vi "ConditioningState.vi"() -> ()   [LabVIEW 2014]
uses:
  ParamsArray.ctl
  state.lvsc/State.ctl
  Licker.lvclass
  Juicer.lvclass
  Acquisition.lvclass
  <vilib>/Utility/error.llb/DialogType.ctl
  Stimulus.lvclass
  state.lvsc/Inputs.ctl
  state.lvsc/Trigger.ctl
  <vilib>/Statechart/Common/IntGuid.ctl
  <vilib>/Statechart/Common/DbgID.ctl
  state.lvsc/StatechartState.ctl
  <vilib>/Utility/file.llb/Read From Spreadsheet File (DBL).vi
  state.lvsc/CompanionDiagram.vi/43/SC Main.vi
  <vilib>/Statechart/Nodes/EventFiring/NI_SC_EventFiringNode.xnode
  state.lvsc
  <vilib>/Statechart/Infrastructure/RTStatechart/RunTime SCN.xnode
  state.lvsc/Outputs.ctl
  <vilib>/Statechart/Common/NI_SC_LVSCCommonFiles.lvlib
panel:
  in  "default pulse duration":dbl
  in  "Local\nDatabase":bool
  in  "Que mail":dbl=500.0
  in  "mail":bool=TRUE
  in  "Reset":bool
  out "error out":errorcluster
  in  "liquid":string(combo)="water"
  in  "Thr":dbl[](array[numeric])=[10.0, 10.0, 10.0, 10.0, 10.0]
  out "Optical traces":waveform(dbl)[](graph)
  in  "Task":dbl[](array[numeric])=[0.0, 0.0, 0.0, 0.0, 0.0]
  out "Licks 2":bool[](array[boolean])
  in  "screen_setup":u16(ring) items=["Default", "1"]
  out "queue#":i32
  in  "Probes":enum16{"Testing", "1-5", "6-10"}(ring)
  in  "Display":bool
  out "Mon params":dbl[][](array[numeric])=[[100.0, 100.0, 0.0, 0.0], [100.0, 100.0, 100.0, 0.0], [100.0, 100.0, 200.0, 0.0], [100.0, 100.0, 300.0, 0.0], [100.0, 100.0, 400.0, 0.0]]
  out "Air":bool[](array[boolean])
  out "CS":bool[](array[boolean])
  out "Active States":T1[][](array[typedef])
  out "Number of Licks":dbl[](array[numeric]) caption="#Licks"
  in  "LICK":bool[](array[boolean])=[FALSE, FALSE, FALSE, FALSE, FALSE]
  out "Elapsed Time":dbl[](array[numeric]) caption="Time"
  out "Rewards Given":dbl[](array[numeric]) caption="#Rew"
  out "Water":bool[](array[boolean])
  out "Licks":bool[](array[boolean])
  out "Sti":i32
  in  "RUN":bool[](array[boolean])=[FALSE, FALSE, FALSE, FALSE, FALSE]
  out "Lick":i32
  out "Acq":i32
  out "Jui":i32
  in  "REC":bool[](array[boolean])=[FALSE, FALSE, FALSE, FALSE, FALSE]
  in  "Stop":bool
  in  "Params":T2={"Mice ID"=[1.0, 1.0, 1.0, 1.0, 1.0], "ExpType"=["Orientation", "Orientation", "Orientation", "Orientation", "Orientation"], "Trial Interval"=[30.0, 30.0, 30.0, 30.0, 30.0], "Pulse Duration"=[158.0, 152.0, 156.0, 167.0, 172.0], "microL_per_pulse"=[6.0, 6.0, 6.0, 6.0, 6.0], "Response Interval"=[1000.0, 1000.0, 1000.0, 1000.0, 1000.0], "Bad Delay"=[180.0, 180.0, 180.0, 180.0, 180.0], "Response Period"=[30.0, 30.0, 30.0, 30.0, 30.0], "liquid_type"="water", "Stimuli"=["", "", "", "", ""], "Rewarded Stimuli"=["", "", "", "", ""], "AirDur"=[400.0, 400.0, 400.0, 400.0, 400.0]} {"AirDur" format="%#_13g"}
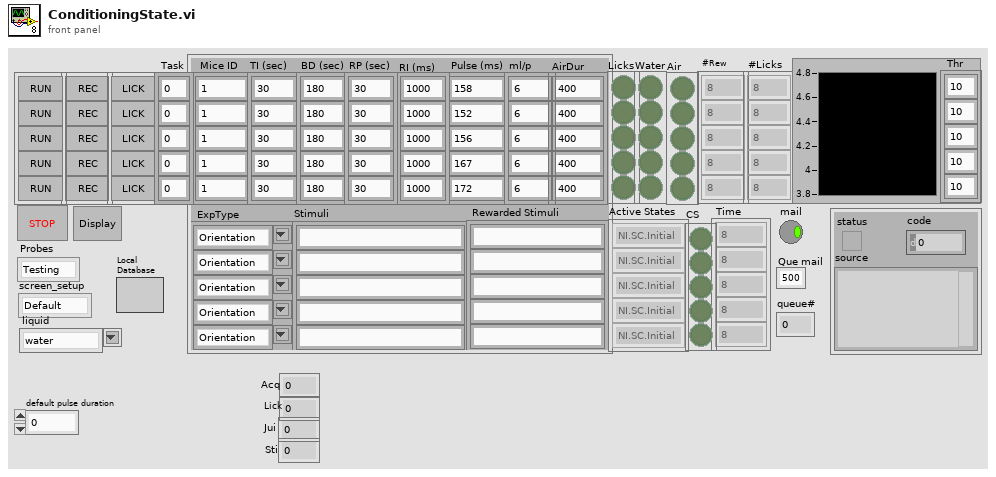
[diagram p1: front panel]
types:
  T1 = typedef "state.lvsc/State.ctl" = enum16{"NI.SC.Initial", "NI.SC.History", "NI.SC.ShallowHistory", "NI.SC.Terminal", "Reward", "Punishment", "Response \nPeriod", "EndTrial", "Start trial"}
  T2 = typedef "ParamsArray.ctl" = cluster{"Mice ID":dbl[], "ExpType":string[], "Trial Interval":dbl[], "Pulse Duration":dbl[], "microL_per_pulse":dbl[], "Response Interval":dbl[], "Bad Delay":dbl[], "Response Period":dbl[], "liquid_type":string, "Stimuli":string[], "Rewarded Stimuli":string[], "AirDur":dbl[]}
  T3 = typedef "DialogType.ctl" = u16
  T4 = typedef "Semaphore RefNum" = refnum<k1>
  T5 = enum16{"air_delivery", "beh_session", "stim_periods", "licks", "liquid_delivery", ""}
  T6 = enum16{"Get Time", "Get Elapsed Time", "Reset Elapsed Time"}
  T7 = typedef "state.lvsc/Inputs.ctl" = cluster{"Acquisition.lvclass":refnum<class "Acquisition.lvclass">, "Stimulus.lvclass":refnum<class "Stimulus.lvclass">, "Juicer.lvclass":refnum<class "Juicer.lvclass">, "Index":dbl, "error in (no error)":errorcluster, "Lick":bool, "State":string}
  T8 = typedef "state.lvsc/Trigger.ctl" = enum16{"NULL", "Lick", "Exit"}
  T9 = typedef "state.lvsc/StatechartState.ctl" = T1[]
  T10 = typedef "NI_SC_LVSCCommonFiles.lvlib/IntGuid.ctl" = cluster{"Data1":u32, "Data2":u16, "Data3":u16, "Data4":u8, "Data5":u8, "Data6":u8, "Data11":u8, "Data9":u8, "Data10":u8, "Data8":u8, "Data7":u8}
  T11 = typedef "NI_SC_LVSCCommonFiles.lvlib/DbgID.ctl" = cluster{"VIRef":u32, "IntGUID":T10}
  T12 = typedef "state.lvsc/Outputs.ctl" = cluster{"Stimulus.lvclass":refnum<class "Stimulus.lvclass">, "error out":errorcluster, "State":string, "Index":dbl, "Correct Response":bool}
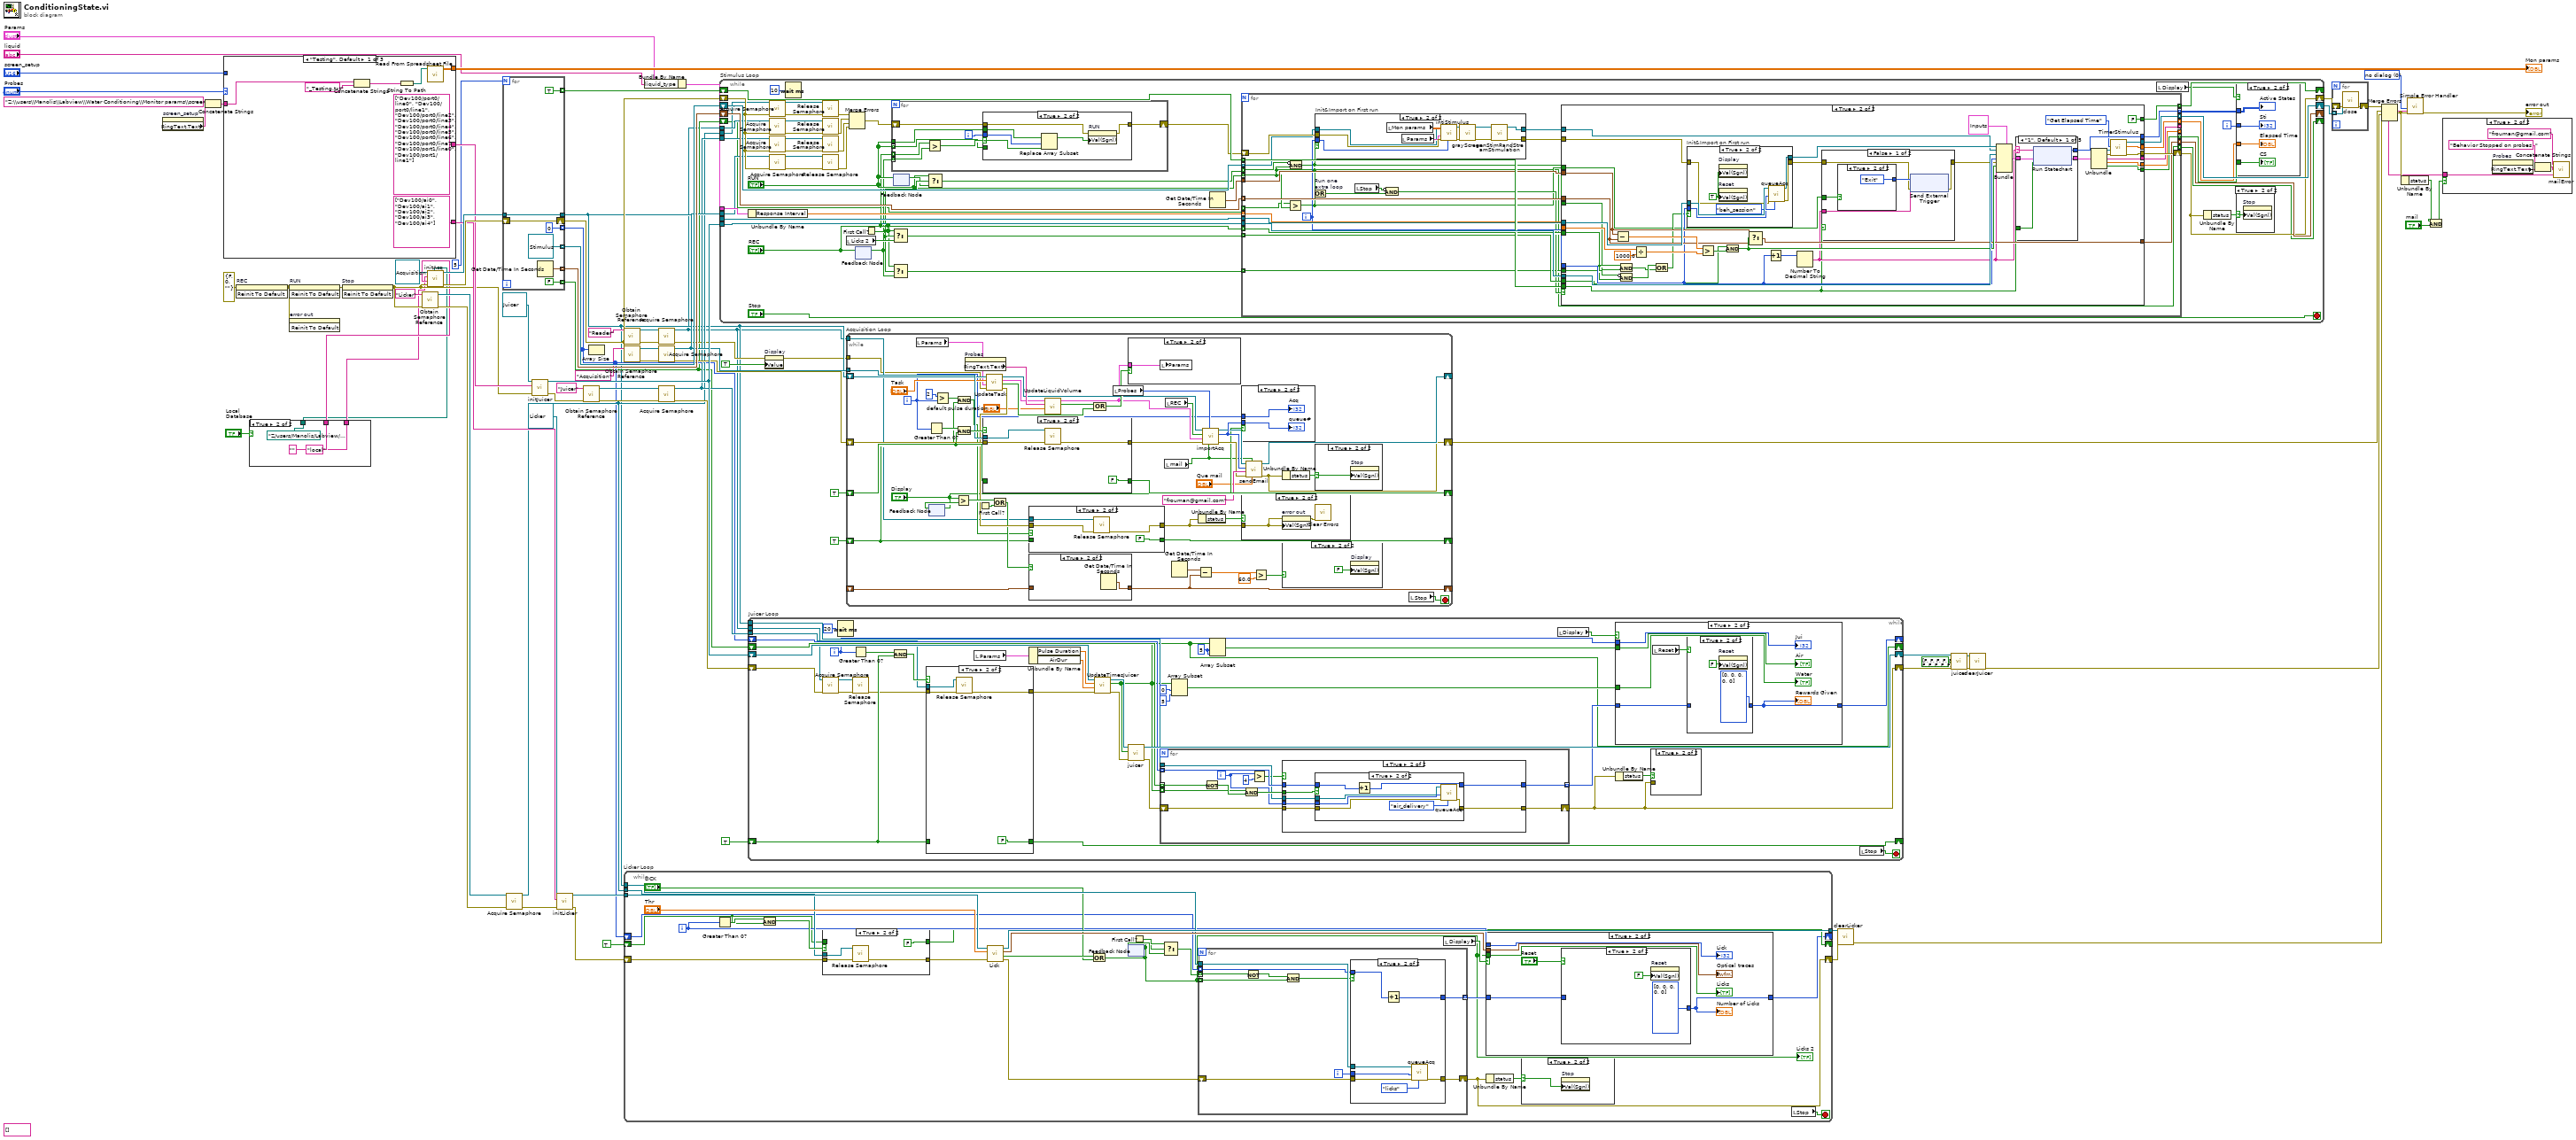
[diagram p0: block diagram]
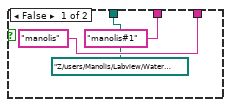
[diagram p2: hidden frame]
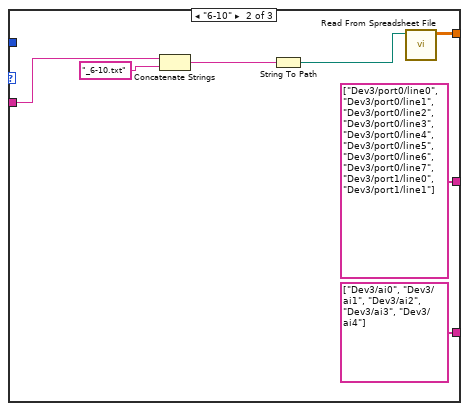
[diagram p4: hidden frame]
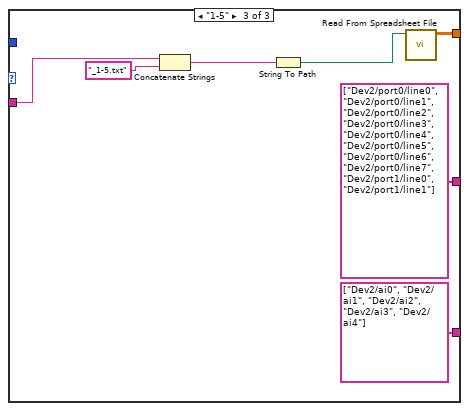
[diagram p5: hidden frame]
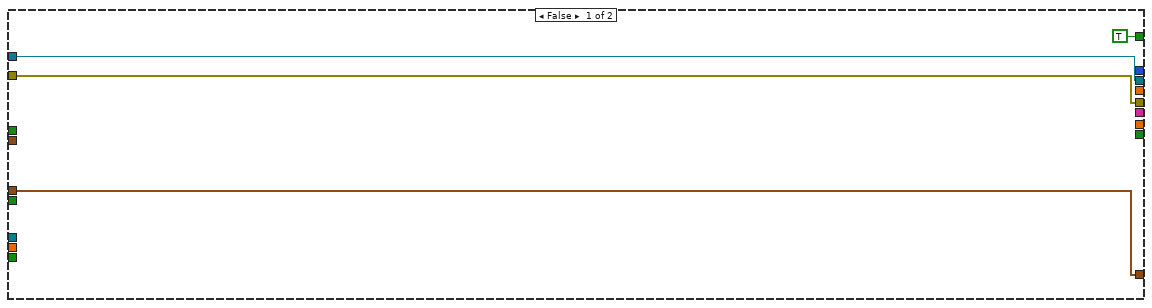
[diagram p10: hidden frame]
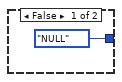
[diagram p11: hidden frame]
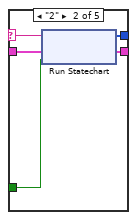
[diagram p14: hidden frame]
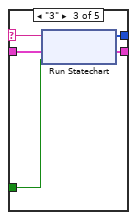
[diagram p15: hidden frame]
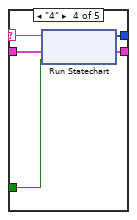
[diagram p16: hidden frame]
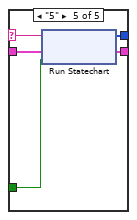
[diagram p17: hidden frame]
diagram:
  (unwired) string[] [] ("Mail addresses")
  w19 = T3 0 items=["no dialog", "OK message", "continue or stop message", "OK message + warnings", "continue/stop + warnings"] ("type of dialog (OK msg:1)")
  n1 = property on="screen_setup" class="Ring (strict)"() -> ("RingText.Text"=w49:string)  [unwired: 2 in, 2 out]
  n2 = Concatenate Strings("Z:\\users\\Manolis\\Labview\\Water Conditioning\\Monitor params\\screen_" ("file path (dialog if empty)"), w49) -> (w48:string)
  n3 = case shown="\"Testing\", Default" "Probes" {
    tunnel: [w83 w90 w97] -> w61
    tunnel: [string[] ["Dev100/port0/line0", "Dev100/port0/line1", "Dev100/port0/line2", "Dev100/port0/line3", "Dev100/port0/line4", "Dev100/port0/line5", "Dev100/port0/line6", "Dev100/port0/line7", "Dev100/port1/line0", "Dev100/port1/line1"] ("Lines") string[] ["Dev3/port0/line0", "Dev3/port0/line1", "Dev3/port0/line2", "Dev3/port0/line3", "Dev3/port0/line4", "Dev3/port0/line5", "Dev3/port0/line6", "Dev3/port0/line7", "Dev3/port1/line0", "Dev3/port1/line1"] ("Lines") string[] ["Dev2/port0/line0", "Dev2/port0/line1", "Dev2/port0/line2", "Dev2/port0/line3", "Dev2/port0/line4", "Dev2/port0/line5", "Dev2/port0/line6", "Dev2/port0/line7", "Dev2/port1/line0", "Dev2/port1/line1"] ("Lines")] -> w60
    tunnel: [string[] ["Dev100/ai0", "Dev100/ai1", "Dev100/ai2", "Dev100/ai3", "Dev100/ai4"] ("Lines") string[] ["Dev3/ai0", "Dev3/ai1", "Dev3/ai2", "Dev3/ai3", "Dev3/ai4"] ("Lines") string[] ["Dev2/ai0", "Dev2/ai1", "Dev2/ai2", "Dev2/ai3", "Dev2/ai4"] ("Lines")] -> w59
    tunnel: "screen_setup" -> [_ _ _]
    tunnel: w48 -> [w85 w91 w98]
    frame "Testing", Default {
      n4 = Concatenate Strings(w85, "_Testing.txt" ("string")) -> (w86:string)
      n5 = String To Path(string=w86) -> (path=w87:path)
      n6 = call-poly <vilib>:"Read From Spreadsheet File.vi"("file path (dialog if empty)"=w87) -> ("all rows"=w83:dbl[][])  [unwired: 6 in, 4 out]
    }
    frame "6-10" {
      n7 = Concatenate Strings(w91, "_6-10.txt" ("string")) -> (w93:string)
      n8 = String To Path(string=w93) -> (path=w94:path)
      n9 = call-poly <vilib>:"Read From Spreadsheet File.vi"("file path (dialog if empty)"=w94) -> ("all rows"=w90:dbl[][])  [unwired: 6 in, 4 out]
    }
    frame "1-5" {
      n10 = Concatenate Strings(w98, "_1-5.txt" ("string")) -> (w100:string)
      n11 = String To Path(string=w100) -> (path=w101:path)
      n12 = call-poly <vilib>:"Read From Spreadsheet File.vi"("file path (dialog if empty)"=w101) -> ("all rows"=w97:dbl[][])  [unwired: 6 in, 4 out]
    }
  }
  "Mon params" <- w61
  n13 = invoke on="REC" class="Arr (strict)" method="Reinit To Default"(error in=errorcluster {"status"=FALSE, "code"=0, "source"=""} ("error in (no error)")) -> (error out=w12:errorcluster)  [unwired: 2 in, 2 out]
  n14 = case shown="True" "Local\nDatabase" {
    tunnel: ["manolis#1" ("password") "" ("password")] -> w4
    tunnel: ["manolis" ("userID") "local" ("userID")] -> w3
    tunnel: [path "Z:/users/Manolis/Labview/Water Conditioning/sessions_remote.dsn" ("Session") path "Z:/users/Manolis/Labview/Water Conditioning/sessions_loca.dsn" ("Session")] -> w2
    frame False {
    }
    frame True {
    }
  }
  n15 = invoke on="RUN" class="Arr (strict)" method="Reinit To Default"(error in=w12) -> (error out=w71:errorcluster)  [unwired: 2 in, 2 out]
  n16 = invoke on="error out" class="Clust (strict)" method="Reinit To Default"(error in=w12) -> ()  [unwired: 2 in, 3 out]
  n17 = invoke on="Stop" class="Bool (strict)" method="Reinit To Default"(error in=w71) -> (error out=w29:errorcluster)  [unwired: 2 in, 2 out]
  n18 = call <vilib>:"Obtain Semaphore Reference.vi"("error in (no error)"=w29, "name (unnamed)"="Licker") -> ("error out"=w32:errorcluster, "semaphore"=w30:T4)  [unwired: 3 in, 1 out]
  n19 = call-dynamic "initAcq.vi"("Session"=w2, "error in (no error)"=w29, "password"=w4, "userID"=w3, "Acquisition in"=refnum<class "Acquisition.lvclass"> refnum ("Acquisition.lvclass")) -> ("error out"=w63:errorcluster, "Acquisition out"=w64:refnum<class "Acquisition.lvclass">)  [unwired: 5 in]
  n20 = for {
    N: 5 -> [_]
    tunnel: [refnum<class "Stimulus.lvclass"> refnum ("Stimulus.lvclass")] -> w69 mode=indexing
    shift-right: [w110] -> w34
    shift-left: w63 -> [w110]
    tunnel: [TRUE] -> w65 mode=indexing
    tunnel: [FALSE] -> w17 mode=indexing
    tunnel: [0] -> w22 mode=indexing
    tunnel: [w113] -> w57 mode=indexing
    tunnel: w64 -> [w112]
    tunnel: [w112] -> w16
    n21 = Get Date/Time In Seconds() -> (seconds since 1Jan1904=w113:timestamp)
  }
  n22 = call <vilib>:"Acquire Semaphore.vi"("error in (no error)"=w32, "semaphore"=w30) -> ("error out"=w28:errorcluster, "semaphore out"=w25:T4)  [unwired: 3 in, 1 out]
  n23 = call-dynamic "initJuicer.vi"("error in (no error)"=w29, "Lines"=w60, "Juicer in"=refnum<class "Juicer.lvclass"> refnum ("Juicer.lvclass")) -> ("error out"=w41:errorcluster, "Juicer out"=w72:refnum<class "Juicer.lvclass">)  [unwired: 7 in]
  n24 = call-dynamic "initLicker.vi"("error in (no error)"=w28, "Lines"=w59, "Licker in"=refnum<class "Licker.lvclass"> refnum ("Licker.lvclass")) -> ("error out"=w78:errorcluster, "Licker out"=w80:refnum<class "Licker.lvclass">)  [unwired: 7 in]
  n25 = call <vilib>:"Obtain Semaphore Reference.vi"("error in (no error)"=w41, "name (unnamed)"="Juicer") -> ("error out"=w44:errorcluster, "semaphore"=w42:T4)  [unwired: 3 in, 1 out]
  n26 = Array Size(array=w22) -> ()  [unwired: 1 out]
  n27 = call <vilib>:"Obtain Semaphore Reference.vi"("error in (no error)"=w34, "name (unnamed)"="Reader") -> ("error out"=w45:errorcluster, "semaphore"=w47:T4)  [unwired: 3 in, 1 out]
  n28 = call <vilib>:"Obtain Semaphore Reference.vi"("error in (no error)"=w34, "name (unnamed)"="Acquisition") -> ("error out"=w37:errorcluster, "semaphore"=w35:T4)  [unwired: 3 in, 1 out]
  n29 = while "Licker Loop" {
    tunnel: w80 -> [w142]
    tunnel: [w141] -> w79
    shift-right: [w117] -> _
    shift-left: w22 -> [w123]
    tunnel: w16 -> [w135]
    tunnel: w25 -> [w129]
    shift-right: [w125] -> _
    shift-left: TRUE -> [w124]
    shift-right: [w118] -> w76
    shift-left: w78 -> [w127]
    i -> [w128]
    stop <- w143 stop-if-true
    n30 = Greater Than 0?(x=w128) -> (x > 0?=w130:bool)
    n31 = And(x=w130, y=w124) -> (x .and. y?=w131:bool)
    n32 = case shown="True" w131 {
      tunnel: [w145 FALSE] -> w125
      tunnel: w127 -> [w144 w148]
      tunnel: w124 -> [w145 _]
      tunnel: w129 -> [_ w147]
      tunnel: [w144 w146] -> w126
      frame False {
      }
      frame True {
        n33 = call <vilib>:"Release Semaphore.vi"("error in (no error)"=w148, "semaphore"=w147) -> ("error out"=w146:errorcluster)  [unwired: 4 in, 1 out]
      }
    }
    n34 = call-dynamic "Lick.vi"("error in (no error)"=w126, "% decrease Thr"="Thr", "Licker in"=w142) -> ("error out"=w138:errorcluster, "Lick?"=w136:bool[], "data"=w140:waveform(dbl)[], "Licker out"=w141:refnum<class "Licker.lvclass">)  [unwired: 5 in]
    n35 = Or(x=w136, y="LICK") -> (x .or. y?=w121:bool[])
    "Licks 2" <- w121
    n36 = feedback-in #1(w121) -> ()
    n37 = feedback #1() -> (w122:bool[])  [unwired: 1 in]
    n38 = First Call?() -> (First Call?: T/F=w120:bool)
    n39 = Select(t=w121, s=w120, f=w122) -> (s? t:f=w119:bool[])
    n40 = for {
      tunnel: w121 -> [w166] mode=indexing
      shift-right: [w169] -> w118
      shift-left: w138 -> [w170]
      tunnel: w119 -> [w165] mode=indexing
      tunnel: w123 -> [w162] mode=indexing
      tunnel: [w161] -> w132 mode=indexing
      tunnel: w135 -> [w168]
      i -> [w167]
      n41 = Not(x=w165) -> (.not. x?=w164:bool)
      n42 = And(x=w164, y=w166) -> (x .and. y?=w163:bool)
      n43 = case shown="True" w163 {
        tunnel: w167 -> [_ w176]
        tunnel: w170 -> [w172 w179]
        tunnel: [w172 w178] -> w169
        tunnel: w168 -> [_ w177]
        tunnel: w162 -> [w171 w175]
        tunnel: [w171 w174] -> w161
        frame False {
        }
        frame True {
          n44 = Increment(x=w175) -> (x+1=w174:i32)
          n45 = call-dynamic "queueAcq.vi"("table"=T5."licks", "error in (no error)"=w179, "Window Number (0...15)"=w176, "Acquisition in"=w177) -> ("error out"=w178:errorcluster)  [unwired: 5 in, 2 out]
        }
      }
    }
    n46 = local read "Display"() -> (w133:bool)
    n47 = case shown="True" w133 {
      tunnel: w140 -> [_ w156]
      tunnel: w128 -> [_ w155]
      tunnel: w132 -> [w150 w153]
      tunnel: w121 -> [_ w154]
      tunnel: [w150 w152] -> w117
      frame False {
      }
      frame True {
        n48 = case shown="True" "Reset" {
          tunnel: w153 -> [w157 _]
          tunnel: [w157 i32[] [0, 0, 0, 0, 0]] -> w152
          frame False {
          }
          frame True {
            n49 = property on="Reset" class="Bool (strict)"("Val(Sgnl)"=FALSE ("Value (Signaling)")) -> ()  [unwired: 2 in, 2 out]
          }
        }
        "Number of Licks" <- w152
        "Optical traces" <- w156
        "Lick" <- w155
        "Licks" <- w154
      }
    }
    n50 = Unbundle By Name(w118) -> ("status"=w137:bool)
    n51 = case shown="True" w137 {
      selector: w137 -> [_ w160]
      frame False {
      }
      frame True {
        n52 = property on="Stop" class="Bool (strict)"("Val(Sgnl)"=w160) -> ()  [unwired: 2 in, 2 out]
      }
    }
    n53 = local read "Stop"() -> (w143:bool)
  }
  n54 = Bundle By Name(cluster="Params", "liquid_type"="liquid") -> (w14:T2)
  n55 = call <vilib>:"Acquire Semaphore.vi"("error in (no error)"=w45, "semaphore"=w47) -> ("error out"=w23:errorcluster, "semaphore out"=w11:T4)  [unwired: 3 in, 1 out]
  n56 = call <vilib>:"Acquire Semaphore.vi"("error in (no error)"=w37, "semaphore"=w35) -> ("error out"=w33:errorcluster, "semaphore out"=w27:T4)  [unwired: 3 in, 1 out]
  n57 = call <vilib>:"Acquire Semaphore.vi"("error in (no error)"=w44, "semaphore"=w42) -> ("error out"=w40:errorcluster, "semaphore out"=w26:T4)  [unwired: 3 in, 1 out]
  n58 = while "Stimulus Loop" {
    tunnel: w72 -> [w229]
    shift-right: [w224] -> w68
    shift-left: w69 -> [w218]
    tunnel: w16 -> [w226]
    shift-right: [w225] -> _
    shift-left: w65 -> [w192]
    shift-right: [w222] -> _
    shift-left: w57 -> [w217]
    tunnel: w14 -> [w221]
    tunnel: w27 -> [w198]
    tunnel: w26 -> [w197]
    tunnel: w11 -> [w196]
    tunnel: w25 -> [w195]
    shift-right: [w182] -> w67
    shift-left: w34 -> [w203]
    shift-right: [w181] -> _
    shift-left: w17 -> [w180]
    i -> [w213]
    stop <- "Stop" stop-if-true
    n59 = Unbundle By Name(w221) -> ("Response Interval"=w219:dbl[])
    n60 = call <vilib>:"Acquire Semaphore.vi"("error in (no error)"=w203, "semaphore"=w195) -> ("error out"=w210:errorcluster, "semaphore out"=w211:T4)  [unwired: 3 in, 1 out]
    n61 = call <vilib>:"Acquire Semaphore.vi"("error in (no error)"=w203, "semaphore"=w196) -> ("error out"=w209:errorcluster, "semaphore out"=w208:T4)  [unwired: 3 in, 1 out]
    n62 = call <vilib>:"Acquire Semaphore.vi"("error in (no error)"=w203, "semaphore"=w197) -> ("error out"=w206:errorcluster, "semaphore out"=w207:T4)  [unwired: 3 in, 1 out]
    n63 = call <vilib>:"Acquire Semaphore.vi"("error in (no error)"=w203, "semaphore"=w198) -> ("error out"=w205:errorcluster, "semaphore out"=w204:T4)  [unwired: 3 in, 1 out]
    n64 = Wait (ms)(milliseconds to wait=u32 10) -> ()  [unwired: 1 out]
    n65 = call <vilib>:"Release Semaphore.vi"("error in (no error)"=w210, "semaphore"=w211) -> ("error out"=w202:errorcluster)  [unwired: 4 in, 1 out]
    n66 = call <vilib>:"Release Semaphore.vi"("error in (no error)"=w209, "semaphore"=w208) -> ("error out"=w201:errorcluster)  [unwired: 4 in, 1 out]
    n67 = call <vilib>:"Release Semaphore.vi"("error in (no error)"=w206, "semaphore"=w207) -> ("error out"=w200:errorcluster)  [unwired: 4 in, 1 out]
    n68 = call <vilib>:"Release Semaphore.vi"("error in (no error)"=w205, "semaphore"=w204) -> ("error out"=w199:errorcluster)  [unwired: 4 in, 1 out]
    n69 = local read "Licks 2"() -> (w191:bool[])
    n70 = Merge Errors(w202, w201, w200, w199) -> (w184:errorcluster)
    n71 = feedback #2() -> (w185:bool[])  [unwired: 1 in]
    n72 = feedback-in #2("REC") -> ()
    n73 = First Call?() -> (First Call?: T/F=w190:bool)
    n74 = for {
      tunnel: "RUN" -> [w236] mode=indexing
      tunnel: "RUN" -> [w235]
      tunnel: "REC" -> [w233] mode=indexing
      tunnel: w185 -> [w232] mode=indexing
      shift-right: [w230] -> w183
      shift-left: w184 -> [w231]
      i -> [w234]
      n75 = Greater?(x=w233, y=w232) -> (0:w237:bool)
      n76 = case shown="True" w237 {
        selector: w237 -> [_ w242]
        tunnel: w236 -> [_ _]
        tunnel: w235 -> [_ w244]
        tunnel: w234 -> [_ w243]
        tunnel: w231 -> [w238 w240]
        tunnel: [w238 w239] -> w230
        frame False {
        }
        frame True {
          n77 = Replace Array Subset(array=w244, new element=w242, index=w243) -> (w241:bool[])
          n78 = property on="RUN" class="Arr (strict)"(error in=w240, "Val(Sgnl)"=w241) -> (error out=w239:errorcluster)  [unwired: 1 in, 1 out]
        }
      }
    }
    n79 = Select(t="REC", s=w190, f=w191) -> (s? t:f=w189:bool[])
    n80 = Select(t="REC", s=w190, f=w185) -> (s? t:f=w193:bool[])
    n81 = feedback-in #3("RUN") -> ()
    n82 = feedback #3() -> (w188:bool[])  [unwired: 1 in]
    n83 = Select(t="RUN", s=w190, f=w188) -> (s? t:f=w194:bool[])
    n84 = Get Date/Time In Seconds() -> (seconds since 1Jan1904=w223:timestamp)
    n85 = for {
      tunnel: "RUN" -> [w251] mode=indexing
      tunnel: w229 -> [w280]
      shift-right: [w279] -> w182
      shift-left: w183 -> [w264]
      tunnel: w226 -> [w269]
      tunnel: w192 -> [w278] mode=indexing
      tunnel: [w277] -> w225 mode=indexing
      tunnel: [w276] -> w214 mode=indexing
      tunnel: [w275] -> w215 mode=indexing
      tunnel: [w274] -> _ mode=indexing
      tunnel: [w273] -> _ mode=indexing
      tunnel: w218 -> [w262] mode=indexing
      tunnel: [w272] -> w224 mode=indexing
      tunnel: [w271] -> w216 mode=indexing
      tunnel: w189 -> [w270] mode=indexing
      tunnel: "REC" -> [w260] mode=indexing
      tunnel: w217 -> [w267] mode=indexing
      tunnel: w223 -> [w268]
      tunnel: [w266] -> w222 mode=indexing
      tunnel: w219 -> [w265] mode=indexing
      tunnel: w194 -> [w258] mode=indexing
      tunnel: w193 -> [w255] mode=indexing
      tunnel: [w251] -> w181 mode=indexing
      tunnel: w180 -> [w250] mode=indexing
      i -> [w259]
      n86 = Greater?(x=w250, y=w251) -> (0:w252:bool)
      n87 = Compound Arithmetic op=AND(invert w258, w251) -> (w254:bool)
      n88 = Or "Run one \nextra loop"(x=w251, y=w252) -> (x .or. y?=w253:bool)
      n89 = case "Init&Import on First run" shown="True" w254 {
        tunnel: [w282 w284] -> w263
        tunnel: w264 -> [w282 w288]
        tunnel: w259 -> [_ w287]
        tunnel: [w281 w289] -> w261
        tunnel: w262 -> [w281 w283]
        frame False {
        }
        frame True {
          n90 = local read "Mon params"() -> (w285:dbl[][])
          n91 = local read "Params"() -> (w286:T2)
          n92 = call-dynamic "intiStimulus.vi"("index"=w287, "error in (no error)"=w288, "Params"=w286, "Monitor parameters"=w285, "Stimulus in"=w283) -> ("error out"=w291:errorcluster, "Stimulus out"=w290:refnum<class "Stimulus.lvclass">)  [unwired: 5 in]
          n93 = call-dynamic "grayScreen.vi"("error in (no error)"=w291, "Stimulus in"=w290) -> ("error out"=w293:errorcluster, "Stimulus out"=w292:refnum<class "Stimulus.lvclass">)  [unwired: 8 in]
          n94 = call-dynamic "genStimRandStreamStimulation.vi"("error in (no error)"=w293, "Stimulus in"=w292) -> ("error out"=w284:errorcluster, "Stimulus out"=w289:refnum<class "Stimulus.lvclass">)  [unwired: 8 in]
        }
      }
      n95 = local read "Stop"() -> (w257:bool)
      n96 = Compound Arithmetic op=AND(invert w257, w253) -> (w256:bool)
      n97 = case shown="True" w256 {
        tunnel: w269 -> [_ w326]
        tunnel: w261 -> [w295 w299]
        tunnel: w280 -> [_ w339]
        tunnel: [w294 w305] -> w279
        tunnel: [w295 w313] -> w272
        tunnel: w263 -> [w294 w324]
        tunnel: w259 -> [_ w314]
        tunnel: w278 -> [_ w302]
        tunnel: [TRUE FALSE] -> w277
        tunnel: [_ w337] -> w276
        tunnel: [_ w336] -> w275
        tunnel: [_ w330] -> w274
        tunnel: [_ w329] -> w273
        tunnel: [_ w312] -> w271
        tunnel: w270 -> [_ w300]
        tunnel: w268 -> [_ w316]
        tunnel: w267 -> [w296 w317]
        tunnel: [w296 w315] -> w266
        tunnel: w265 -> [_ w319]
        tunnel: w260 -> [_ w308]
        tunnel: w255 -> [_ w311]
        tunnel: w254 -> [_ w307]
        tunnel: w252 -> [_ w298]
        frame False {
        }
        frame True {
          n98 = Subtract(x=w316, y=w317) -> (x-y=w320:dbl)
          n99 = And(x=w308, y=w307) -> (x .and. y?=w309:bool)
          n100 = Compound Arithmetic op=AND(invert w311, w308) -> (w310:bool)
          n101 = Divide(x=w319, y=1000.0) -> (x/y=w323:dbl)
          n102 = Or(x=w310, y=w309) -> (x .or. y?=w306:bool)
          n103 = case "Init&Import on First run" shown="True" w306 {
            tunnel: [w364 w372] -> w325
            tunnel: [w365 w371] -> w303
            tunnel: w326 -> [w364 w370]
            tunnel: w324 -> [w365 w367]
            tunnel: w314 -> [_ w368]
            frame False {
            }
            frame True {
              w366 = TRUE ("Value (Signaling)")
              n104 = property on="Display" class="Bool (strict)"("Val(Sgnl)"=w366) -> ()  [unwired: 2 in, 2 out]
              n105 = property on="Reset" class="Bool (strict)"("Val(Sgnl)"=w366) -> ()  [unwired: 2 in, 2 out]
              n106 = call-dynamic "queueAcq.vi"("table"=T5."beh_session", "error in (no error)"=w367, "Window Number (0...15)"=w368, "Acquisition in"=w370) -> ("error out"=w371:errorcluster, "Acquisition out"=w372:refnum<class "Acquisition.lvclass">)  [unwired: 5 in, 1 out]
            }
          }
          n107 = Greater?(x=w320, y=w323) -> (0:w321:bool)
          n108 = And(x=w300, y=w321) -> (x .and. y?=w318:bool)
          n109 = Select(t=w316, s=w318, f=w317) -> (s? t:f=w315:timestamp)
          n110 = Increment(x=w314) -> (x+1=w332:i32)
          n111 = Number To Decimal String(number=w332) -> (decimal integer string=w304:string)  [unwired: 1 in]
          n112 = case shown="False" w302 {
            tunnel: w304 -> [w343 _]
            tunnel: w303 -> [w342 w363]
            tunnel: [w341 w363] -> w301
            tunnel: w298 -> [w340 _]
            frame False {
              n113 = case shown="True" w340 {
                tunnel: [Trigger."NULL" ("Trigger") Trigger."Exit" ("Trigger")] -> w344
                frame False {
                }
                frame True {
                }
              }
              n114 = xnode "Send External Trigger"("Instance Name"=w343, "Trigger"=w344, "error in (no error)"=w342) -> ("error out"=w341:errorcluster)  [unwired: 1 out]
            }
            frame True {
            }
          }
          n115 = Bundle(cluster=T7 {"Acquisition.lvclass"=refnum, "Stimulus.lvclass"=refnum, "Juicer.lvclass"=refnum, "Index"=0.0, "error in (no error)"={"status"=FALSE, "code"=0, "source"=""}, "Lick"=FALSE, "State"=""} ("Inputs"), "Acquisition.lvclass"=w325, "Stimulus.lvclass"=w299, "Juicer.lvclass"=w339, "Index"=w314, "error in (no error)"=w301, "Lick"=w318, "State"=w304) -> (w333:T7)
          n116 = case shown="\"1\", Default" w304 {
            selector: w304 -> [w375 w433 w492 w551 w610]
            tunnel: [w377 w436 w495 w554 w613] -> w335
            tunnel: w333 -> [w376 w435 w494 w553 w612]
            tunnel: w302 -> [w373 w434 w493 w552 w611]
            tunnel: [w374 w432 w491 w550 w609] -> w337
            frame "1", Default {
              n117 = xnode "Run Statechart"("Init?"=w373, "Inputs"=w376, "Instance Name"=w375) -> ("Outputs"=w377:T12, "Active States"=w374:T9)  [unwired: 1 out]
            }
            frame "2" {
              n118 = xnode "Run Statechart"("Init?"=w434, "Inputs"=w435, "Instance Name"=w433) -> ("Outputs"=w436:T12, "Active States"=w432:T9)  [unwired: 1 out]
            }
            frame "3" {
              n119 = xnode "Run Statechart"("Init?"=w493, "Inputs"=w494, "Instance Name"=w492) -> ("Outputs"=w495:T12, "Active States"=w491:T9)  [unwired: 1 out]
            }
            frame "4" {
              n120 = xnode "Run Statechart"("Init?"=w552, "Inputs"=w553, "Instance Name"=w551) -> ("Outputs"=w554:T12, "Active States"=w550:T9)  [unwired: 1 out]
            }
            frame "5" {
              n121 = xnode "Run Statechart"("Init?"=w611, "Inputs"=w612, "Instance Name"=w610) -> ("Outputs"=w613:T12, "Active States"=w609:T9)  [unwired: 1 out]
            }
          }
          n122 = Unbundle(w335) -> ("Stimulus.lvclass"=w328:refnum<class "Stimulus.lvclass">, "error out"=w327:errorcluster, "State"=w330:string, "Index"=w329:dbl, "Correct Response"=w312:bool)
          n123 = call-dynamic "TimerStimulus.vi"("error in (no error)"=w327, "Method"=T6."Get Elapsed Time", "Stimulus in"=w328) -> ("error out"=w305:errorcluster, "Time"=w336:dbl, "Stimulus out"=w313:refnum<class "Stimulus.lvclass">)  [unwired: 5 in, 1 out]
        }
      }
    }
    n124 = local read "Display"() -> (w212:bool)
    n125 = Unbundle By Name(w182) -> ("status"=w227:bool)
    n126 = case shown="True" w212 {
      tunnel: w216 -> [_ w248]
      tunnel: w215 -> [_ w247]
      tunnel: w214 -> [_ w246]
      tunnel: w213 -> [_ w245]
      frame False {
      }
      frame True {
        "CS" <- w248
        "Elapsed Time" <- w247
        "Active States" <- w246
        "Sti" <- w245
      }
    }
    n127 = case shown="True" w227 {
      selector: w227 -> [_ w249]
      frame False {
      }
      frame True {
        n128 = property on="Stop" class="Bool (strict)"("Val(Sgnl)"=w249) -> ()  [unwired: 2 in, 2 out]
      }
    }
  }
  n129 = while "Juicer Loop" {
    shift-right: [w700] -> w56
    shift-left: w72 -> [w701]
    shift-right: [w668] -> _
    shift-left: w22 -> [w695]
    shift-right: [w670] -> _
    shift-left: w17 -> [w693]
    tunnel: w16 -> [w687]
    tunnel: w26 -> [w680]
    shift-right: [w678] -> _
    shift-left: TRUE -> [w677]
    tunnel: w11 -> [w671]
    shift-right: [w669] -> w55
    shift-left: w40 -> [w673]
    i -> [w676]
    stop <- w703 stop-if-true
    w689 = 5 ("index")
    n130 = call <vilib>:"Acquire Semaphore.vi"("error in (no error)"=w673, "semaphore"=w671) -> ("error out"=w674:errorcluster, "semaphore out"=w675:T4)  [unwired: 3 in, 1 out]
    n131 = Wait (ms)(milliseconds to wait=u32 20) -> ()  [unwired: 1 out]
    n132 = call <vilib>:"Release Semaphore.vi"("error in (no error)"=w674, "semaphore"=w675) -> ("error out"=w672:errorcluster)  [unwired: 4 in, 1 out]
    n133 = Greater Than 0?(x=w676) -> (x > 0?=w681:bool)
    n134 = And(x=w681, y=w677) -> (x .and. y?=w682:bool)
    n135 = case shown="True" w682 {
      tunnel: [w705 FALSE] -> w678
      tunnel: w672 -> [w704 w708]
      tunnel: w677 -> [w705 _]
      tunnel: w680 -> [_ w707]
      tunnel: [w704 w706] -> w679
      frame False {
      }
      frame True {
        n136 = call <vilib>:"Release Semaphore.vi"("error in (no error)"=w708, "semaphore"=w707) -> ("error out"=w706:errorcluster)  [unwired: 4 in, 1 out]
      }
    }
    n137 = local read "Params"() -> (w685:T2)
    n138 = Unbundle By Name(w685) -> ("Pulse Duration"=w684:dbl[], "AirDur"=w686:dbl[])
    n139 = call-dynamic "UpdateTimesJuicer.vi"("error in (no error)"=w679, "Air Duration"=w686, "Pulse Duration"=w684, "Juicer in"=w701) -> ("error out"=w699:errorcluster, "Juice"=w670:bool[], "Juicer out"=w702:refnum<class "Juicer.lvclass">)  [unwired: 2 in, 3 out]
    n140 = call-dynamic "juicer.vi"("error in (no error)"=w699, "data"=w670, "Juicer in"=w702) -> ("error out"=w698:errorcluster, "Juicer out"=w700:refnum<class "Juicer.lvclass">)  [unwired: 7 in]
    n141 = for {
      tunnel: w670 -> [w729] mode=indexing
      shift-right: [w727] -> w669
      shift-left: w698 -> [w728]
      tunnel: w695 -> [w726] mode=indexing
      tunnel: [w725] -> w694 mode=indexing
      tunnel: w693 -> [w724] mode=indexing
      tunnel: w687 -> [w723]
      i -> [w720]
      n142 = Not(x=w724) -> (.not. x?=w730:bool)
      n143 = And(x=w729, y=w730) -> (x .and. y?=w731:bool)
      n144 = Greater?(x=w720, y=4) -> (0:w721:bool)
      n145 = case shown="True" w721 {
        tunnel: w731 -> [w738 w754]
        tunnel: w728 -> [w737 w753]
        tunnel: [w736 w752] -> w727
        tunnel: w726 -> [w735 w751]
        tunnel: [w734 w750] -> w725
        tunnel: w720 -> [w733 w749]
        tunnel: w723 -> [w732 w748]
        frame False {
          n146 = case shown="True" w738 {
            tunnel: w733 -> [_ w747]
            tunnel: w737 -> [w740 w746]
            tunnel: [w740 w745] -> w736
            tunnel: w735 -> [w739 w744]
            tunnel: [w739 w743] -> w734
            tunnel: w732 -> [_ w742]
            frame False {
            }
            frame True {
              n147 = Increment(x=w744) -> (x+1=w743:i32)
              n148 = call-dynamic "queueAcq.vi"("table"=T5."liquid_delivery", "error in (no error)"=w746, "Window Number (0...15)"=w747, "Acquisition in"=w742) -> ("error out"=w745:errorcluster)  [unwired: 5 in, 2 out]
            }
          }
        }
        frame True {
          n149 = case shown="True" w754 {
            tunnel: w749 -> [_ w763]
            tunnel: w753 -> [w756 w762]
            tunnel: [w756 w761] -> w752
            tunnel: w751 -> [w755 w760]
            tunnel: [w755 w759] -> w750
            tunnel: w748 -> [_ w758]
            frame False {
            }
            frame True {
              n150 = Increment(x=w760) -> (x+1=w759:i32)
              n151 = call-dynamic "queueAcq.vi"("table"=T5."air_delivery", "error in (no error)"=w762, "Window Number (0...15)"=w763, "Acquisition in"=w758) -> ("error out"=w761:errorcluster)  [unwired: 5 in, 2 out]
            }
          }
        }
      }
    }
    n152 = Array Subset(array=w670, index=0, length=5) -> (w690:bool[])
    n153 = Array Subset(array=w670, index=w689, length=w689) -> (w688:bool[])
    n154 = local read "Display"() -> (w683:bool)
    n155 = case shown="True" w683 {
      tunnel: w694 -> [w710 w713]
      tunnel: w690 -> [_ w716]
      tunnel: w688 -> [_ w715]
      tunnel: w676 -> [_ w714]
      tunnel: [w710 w712] -> w668
      frame False {
      }
      frame True {
        n156 = local read "Reset"() -> (w711:bool)
        n157 = case shown="True" w711 {
          tunnel: w713 -> [w717 _]
          tunnel: [w717 i32[] [0, 0, 0, 0, 0]] -> w712
          frame False {
          }
          frame True {
            n158 = property on="Reset" class="Bool (strict)"("Val(Sgnl)"=FALSE ("Value (Signaling)")) -> ()  [unwired: 2 in, 2 out]
          }
        }
        "Rewards Given" <- w712
        "Water" <- w716
        "Air" <- w715
        "Jui" <- w714
      }
    }
    n159 = Unbundle By Name(w669) -> ("status"=w696:bool)
    n160 = case shown="True" w696 {
      tunnel: w669 -> [_ _]
      frame False {
      }
      frame True {
      }
    }
    n161 = local read "Stop"() -> (w703:bool)
  }
  n162 = property on="Display" class="Bool (strict)"(error in=w23, "Value"=TRUE ("Display")) -> (error out=w9:errorcluster)  [unwired: 1 in, 1 out]
  n163 = while "Acquisition Loop" {
    shift-right: [w802] -> _
    shift-left: w16 -> [w776]
    shift-right: [w809] -> _
    shift-left: TRUE -> [w806]
    tunnel: w27 -> [w807]
    shift-right: [w800] -> w73
    shift-left: w33 -> [w808]
    tunnel: w11 -> [w772]
    shift-right: [w778] -> _
    shift-left: _ -> [w779]
    shift-right: [w774] -> _
    shift-left: TRUE -> [w773]
    tunnel: w9 -> [w769]
    i -> [w768]
    stop <- w814 stop-if-true
    n164 = local read "Params"() -> (w771:T2)
    n165 = Greater Than 0?(x=w768) -> (x > 0?=w811:bool)
    n166 = feedback #4() -> (w789:bool)  [unwired: 1 in]
    n167 = feedback-in #4("Display") -> ()
    n168 = Greater?(x=2, y=w768) -> (0:w787:bool)
    n169 = Greater?(x="Display", y=w789) -> (0:w790:bool)
    n170 = And(x=w787, y=w773) -> (x .and. y?=w784:bool)
    n171 = And(x=w811, y=w806) -> (x .and. y?=w810:bool)
    n172 = property on="Probes" class="Enum (strict)"() -> ("RingText.Text"=w794:string)  [unwired: 2 in, 2 out]
    n173 = First Call?() -> (First Call?: T/F=w791:bool)
    n174 = case shown="True" w810 {
      tunnel: [w829 FALSE] -> w809
      tunnel: w808 -> [w828 w832]
      tunnel: w806 -> [w829 _]
      tunnel: w807 -> [_ w831]
      tunnel: [w828 w830] -> w777
      frame False {
      }
      frame True {
        n175 = call <vilib>:"Release Semaphore.vi"("error in (no error)"=w832, "semaphore"=w831) -> ("error out"=w830:errorcluster)  [unwired: 4 in, 1 out]
      }
    }
    n176 = call-dynamic "UpdateTask.vi"("error in (no error)"=w769, "Params"=w771, "Task"="Task", "Acquisition in"=w776) -> ("error out"=w788:errorcluster, "Change"=w797:bool, "Params 2"=w793:T2, "Acquisition out"=w775:refnum<class "Acquisition.lvclass">)  [unwired: 4 in]
    n177 = Or(x=w790, y=w791) -> (x .or. y?=w785:bool)
    n178 = case shown="True" w784 {
      tunnel: [w820 FALSE] -> w774
      tunnel: w772 -> [_ w823]
      tunnel: w788 -> [w819 w822]
      tunnel: w773 -> [w820 _]
      tunnel: [w819 w821] -> w799
      frame False {
      }
      frame True {
        n179 = call <vilib>:"Release Semaphore.vi"("error in (no error)"=w822, "semaphore"=w823) -> ("error out"=w821:errorcluster)  [unwired: 4 in, 1 out]
      }
    }
    n180 = case shown="True" w785 {
      tunnel: [w826 w827] -> w778
      tunnel: w779 -> [w826 _]
      frame False {
      }
      frame True {
        n181 = Get Date/Time In Seconds() -> (seconds since 1Jan1904=w827:timestamp)
      }
    }
    n182 = call "UpdateLiquidVolume.vi"("default pulse duration"="default pulse duration", "Ring Text.Text"=w794, "Params"=w793) -> ("Change"=w796:bool, "Params 2"=w770:T2)  [unwired: 7 in]
    n183 = Compound Arithmetic op=OR(w796, w797) -> (w795:bool)
    n184 = local read "Probes"() -> (w812:enum16{"Testing", "1-5", "6-10"})
    n185 = case shown="True" w795 {
      tunnel: w770 -> [_ w818]
      frame False {
      }
      frame True {
        n186 = local write "Params"(w818) -> ()
      }
    }
    n187 = local read "mail"() -> (w765:bool)
    n188 = local read "REC"() -> (w813:bool[])
    n189 = Get Date/Time In Seconds() -> (seconds since 1Jan1904=w780:timestamp)
    n190 = Subtract(x=w780, y=w778) -> (x-y=w781:dbl)
    n191 = Unbundle By Name(w799) -> ("status"=w798:bool)
    n192 = call-dynamic "importAcq.vi"("mail"=w765, "Probes"=w812, "error in (no error)"=w777, "Params"=w770, "REC"=w813, "Acquisition in"=w775) -> ("error out"=w801:errorcluster, "# elements in queue"=w804:i32, "Acquisition out"=w803:refnum<class "Acquisition.lvclass">)  [unwired: 3 in]
    n193 = case shown="True" "Display" {
      tunnel: w804 -> [_ w835]
      tunnel: w768 -> [_ w834]
      frame False {
      }
      frame True {
        "queue#" <- w835
        "Acq" <- w834
      }
    }
    n194 = case shown="True" w798 {
      tunnel: w799 -> [_ w817]
      frame False {
      }
      frame True {
        n195 = property on="error out" class="Clust (strict)"(error in=w817, "Val(Sgnl)"=w817) -> (error out=w816:errorcluster)  [unwired: 1 in, 1 out]
        n196 = call <vilib>:"Clear Errors.vi"("error in (no error)"=w816) -> ()  [unwired: 5 in, 2 out]
      }
    }
    n197 = call-dynamic "sendEmail.vi"("Queue limit"="Que mail", "Mail"=w765, "error in (no error)"=w801, "Recipient's Email Address Address"="frouman@gmail.com", "Queue Length"=w804, "Acquisition in"=w803) -> ("error out"=w800:errorcluster, "Acquisition out"=w802:refnum<class "Acquisition.lvclass">)  [unwired: 4 in]
    n198 = Greater?(x=w781, y=60.0) -> (0:w783:bool)
    n199 = Unbundle By Name(w800) -> ("status"=w815:bool)
    n200 = case shown="True" w783 {
      frame False {
      }
      frame True {
        n201 = property on="Display" class="Bool (strict)"("Val(Sgnl)"=FALSE ("Value (Signaling)")) -> ()  [unwired: 2 in, 2 out]
      }
    }
    n202 = case shown="True" w815 {
      selector: w815 -> [_ w836]
      frame False {
      }
      frame True {
        n203 = property on="Stop" class="Bool (strict)"("Val(Sgnl)"=w836) -> ()  [unwired: 2 in, 2 out]
      }
    }
    n204 = local read "Stop"() -> (w814:bool)
  }
  n205 = call-dynamic "clearLicker.vi"("error in (no error)"=w76, "Licker in"=w79) -> ("error out"=w75:errorcluster)  [unwired: 8 in, 1 out]
  n206 = call-dynamic "juicer.vi"("error in (no error)"=w55, "data"=bool[] [FALSE, FALSE, FALSE, FALSE, FALSE, FALSE, FALSE, FALSE, FALSE, FALSE], "Juicer in"=w56) -> ("error out"=w54:errorcluster, "Juicer out"=w53:refnum<class "Juicer.lvclass">)  [unwired: 7 in]
  n207 = call-dynamic "clearJuicer.vi"("error in (no error)"=w54, "Juicer in"=w53) -> ("error out"=w74:errorcluster)  [unwired: 8 in, 1 out]
  n208 = for {
    tunnel: w68 -> [w839] mode=indexing
    shift-right: [w837] -> w66
    shift-left: w67 -> [w838]
    n209 = call-dynamic "close.vi"("error in (no error)"=w838, "Stimulus in"=w839) -> ("error out"=w837:errorcluster)  [unwired: 8 in, 1 out]
  }
  n210 = Merge Errors(w66, w73, w74, w75) -> (w20:errorcluster)
  n211 = Unbundle By Name(w20) -> ("status"=w7:bool)
  n212 = call <vilib>:"Simple Error Handler.vi"("type of dialog (OK msg:1)"=w19, "error in (no error)"=w20) -> ("error out"=→"error out":errorcluster, "message"=w18:string)  [unwired: 3 in, 3 out]
  n213 = And(x=w7, y="mail") -> (x .and. y?=w6:bool)
  n214 = case shown="True" w6 {
    tunnel: w18 -> [_ w843]
    frame False {
    }
    frame True {
      n215 = property on="Probes" class="Enum (strict)"() -> ("RingText.Text"=w840:string)  [unwired: 2 in, 2 out]
      n216 = Concatenate Strings("Behavior Stopped on probes  " ("Subject"), w840) -> (w841:string)
      n217 = call "mailError.vi"("Body"=w843, "Subject"=w841, "Recipient's Email Address Address"="frouman@gmail.com") -> ()  [unwired: 1 in]
    }
  }
